vi "Enum_case.vi"() -> ()   [LabVIEW 2017]
panel:
  in  "stop":bool
  out "result":dbl
  in  "b":dbl
  in  "a":dbl
  in  "Enum":enum16{"add", "subtract", "divide", "multiply"}(ring)
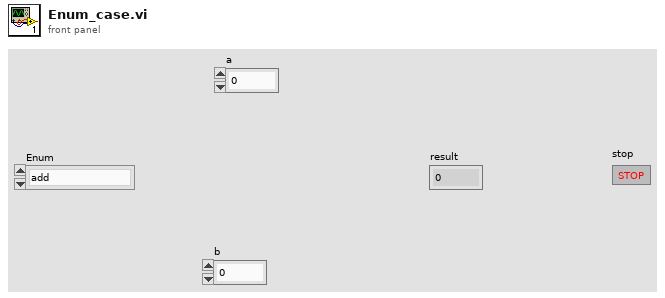
[diagram p1: front panel]
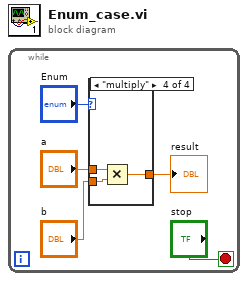
[diagram p0: block diagram]
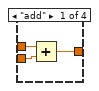
[diagram p2: hidden frame]
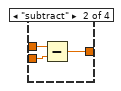
[diagram p3: hidden frame]
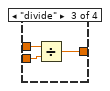
[diagram p4: hidden frame]
diagram:
  n1 = while {
    stop <- "stop" stop-if-true
    n2 = case shown="\"multiply\"" "Enum" {
      tunnel: [w8 w9 w12 w15] -> w1
      tunnel: "a" -> [w7 w11 w14 w17]
      tunnel: "b" -> [w6 w10 w13 w16]
      frame "add" {
        n3 = Add(x=w7, y=w6) -> (x+y=w8:dbl)
      }
      frame "subtract" {
        n4 = Subtract(x=w11, y=w10) -> (x-y=w9:dbl)
      }
      frame "divide" {
        n5 = Divide(x=w14, y=w13) -> (x/y=w12:dbl)
      }
      frame "multiply" {
        n6 = Multiply(x=w17, y=w16) -> (x*y=w15:dbl)
      }
    }
    "result" <- w1
  }
